vi "Do.vi"(8 "error in (no error)":errorcluster, 10 "Actor in":refnum<class "Actor.lvclass">, 11 "Launch Actors Msg":refnum<class "Launch Actors Msg.lvclass">) -> (0 "error out":errorcluster, 2 "Actor out":refnum<class "Actor.lvclass">)   [LabVIEW 2015, in "CS++StartActor.lvlib" / "Launch Actors Msg.lvclass"]
doc: "This VI delivers the message to the actor by calling the appropriate method(s) on the actor."
uses:
  Launch Actors Msg.lvclass
  <vilib>/ActorFramework/Actor/Actor.lvclass
  CS++StartActor/CS++StartActor.lvclass
  Launch Actors Msg.lvclass/Launch Actors Msg.ctl
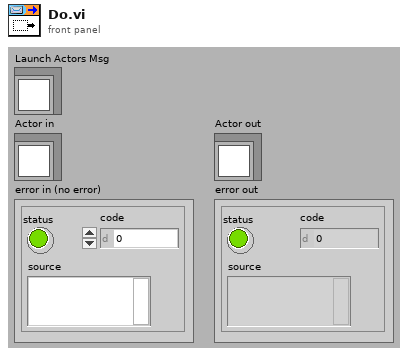
[diagram p1: front panel]
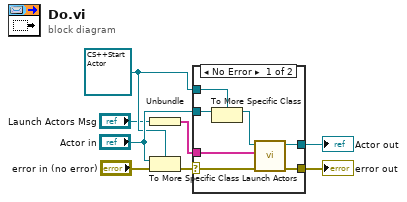
[diagram p0: block diagram]
diagram:
  w3 = refnum<class "CS++StartActor.lvclass"> refnum ("Actor in")
  n1 = Unbundle ("Main-Unbundle")("Launch Actors Msg") -> (w1:string[])
  n2 = To More Specific Class(target class=w3, reference="Actor in", error in="error in (no error)") -> (error out=w7:errorcluster)  [unwired: 1 out]
  n3 = case shown="No Error" w7 {
    selector: w7 -> [w13 w17]
    tunnel: [w15 w17] -> w6
    tunnel: [w14 w16] -> w5
    tunnel: "Actor in" -> [w12 w16]
    tunnel: w3 -> [w11 _]
    tunnel: w1 -> [w9 _]
    frame No Error {
      n4 = To More Specific Class(target class=w11, reference=w12) -> (specific class reference=w10:refnum<class "CS++StartActor.lvclass">)  [unwired: 1 in, 1 out]
      n5 = call "Launch Actors.vi"("error in (no error)"=w13, "Selected Actors"=w9, "CS++StartActor in"=w10) -> ("error out"=w15:errorcluster, "CS++StartActor out"=w14:refnum<class "CS++StartActor.lvclass">)  [unwired: 7 in]
    }
    frame Error {
    }
  }
  "error out" <- w6
  "Actor out" <- w5
